vi "GNSS1-SET-5.vi"(4 "DigNum引用句柄 3":refnum<vi>, 6 "Clust引用句柄 2":refnum<vi>, 7 "DigNum引用句柄":refnum<vi>, 9 "DigNum引用句柄 2":refnum<vi>, 10 "Clust引用句柄":refnum<vi>, 11 "Cluster输入":refnum<vi>) -> (3 "添加的数组":u8[](array[numeric]))   [LabVIEW 2012]
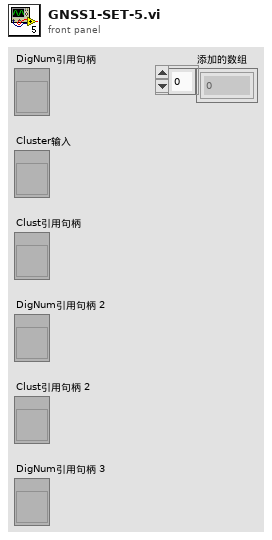
[diagram p1: front panel]
types:
  T1 = cluster{"BD-J2000X轴位置":sgl, "BD-J2000Y轴位置":sgl, "BD-J2000Z轴位置":sgl, "BD-J2000X轴速度":sgl, "BD-J2000Y轴速度":sgl, "BD-J2000Z轴速度":sgl}
  T2 = cluster{"GLOBD-J2000X轴位置":sgl, "GLOBDBD-J2000Y轴位置":sgl, "GLOBD-J2000Z轴位置":sgl, "GLOBD-J2000X轴速度":sgl, "GLOBD-J2000Y轴速度":sgl, "GLOBD-J2000Z轴速度":sgl}
  T3 = cluster{"GPS-J2000X轴位置":sgl, "GPS-J2000Y轴位置":sgl, "GPS-J2000Z轴位置":sgl, "GPS-J2000X轴速度":sgl, "GPS-J2000Y轴速度":sgl, "GPS-J2000Z轴速度":sgl}
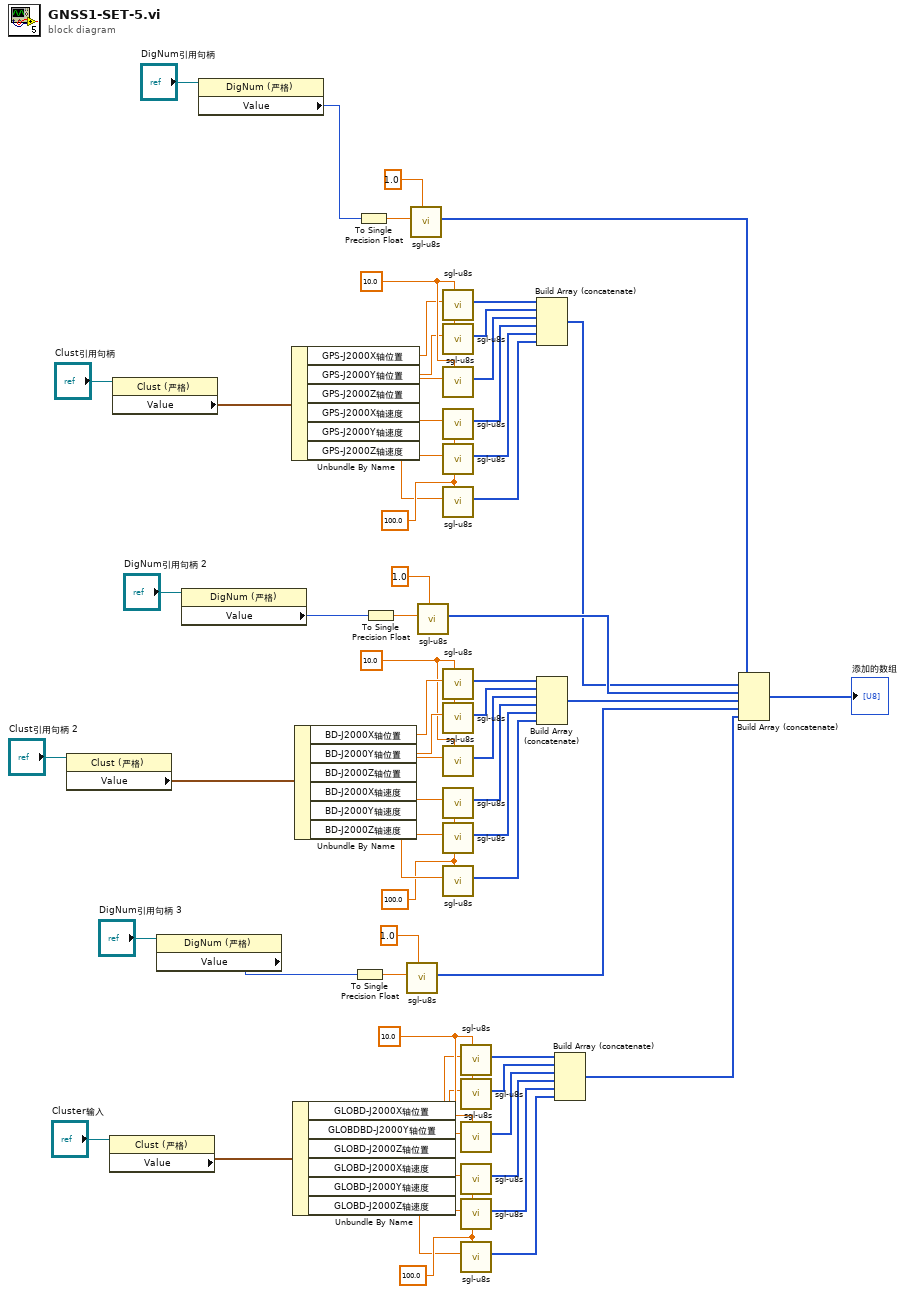
[diagram p0: block diagram]
diagram:
  w58 = sgl 100.0 ("精度")
  w52 = sgl 10.0 ("y")
  w31 = sgl 100.0 ("精度")
  w37 = sgl 10.0 ("y")
  w24 = sgl 100.0 ("精度")
  w18 = sgl 10.0 ("y")
  n1 = property on="属性节点" class="Clust (严格)"(reference="Clust引用句柄 2") -> ("Value"=w59:T1)  [unwired: 1 in, 2 out]
  n2 = property on="属性节点" class="Clust (严格)"(reference="Cluster输入") -> ("Value"=w65:T2)  [unwired: 1 in, 2 out]
  n3 = property on="属性节点" class="Clust (严格)"(reference="Clust引用句柄") -> ("Value"=w25:T3)  [unwired: 1 in, 2 out]
  n4 = property on="属性节点" class="DigNum (严格)"(reference="DigNum引用句柄 3") -> ("Value"=w63:u32)  [unwired: 1 in, 2 out]
  n5 = property on="属性节点" class="DigNum (严格)"(reference="DigNum引用句柄 2") -> ("Value"=w29:u32)  [unwired: 1 in, 2 out]
  n6 = property on="属性节点" class="DigNum (严格)"(reference="DigNum引用句柄") -> ("Value"=w9:u32)  [unwired: 1 in, 2 out]
  n7 = Unbundle By Name(w25) -> ("GPS-J2000X轴位置"=w11:sgl, "GPS-J2000Y轴位置"=w13:sgl, "GPS-J2000Z轴位置"=w14:sgl, "GPS-J2000X轴速度"=w15:sgl, "GPS-J2000Y轴速度"=w16:sgl, "GPS-J2000Z轴速度"=w17:sgl)
  n8 = Unbundle By Name(w65) -> ("GLOBD-J2000X轴位置"=w45:sgl, "GLOBDBD-J2000Y轴位置"=w47:sgl, "GLOBD-J2000Z轴位置"=w48:sgl, "GLOBD-J2000X轴速度"=w49:sgl, "GLOBD-J2000Y轴速度"=w50:sgl, "GLOBD-J2000Z轴速度"=w51:sgl)
  n9 = Unbundle By Name(w59) -> ("BD-J2000X轴位置"=w44:sgl, "BD-J2000Y轴位置"=w42:sgl, "BD-J2000Z轴位置"=w41:sgl, "BD-J2000X轴速度"=w40:sgl, "BD-J2000Y轴速度"=w39:sgl, "BD-J2000Z轴速度"=w38:sgl)
  n10 = To Single Precision Float(number=w63) -> (single precision float=w62:sgl)
  n11 = To Single Precision Float(number=w9) -> (single precision float=w8:sgl)
  n12 = To Single Precision Float(number=w29) -> (single precision float=w27:sgl)
  n13 = call "sgl-u8s.vi"("输入sgl"=w62, "精度"=sgl 1.0) -> ("u8s"=w64:u8[])  [unwired: 8 in]
  n14 = call "sgl-u8s.vi"("输入sgl"=w8, "精度"=sgl 1.0) -> ("u8s"=w10:u8[])  [unwired: 8 in]
  n15 = call "sgl-u8s.vi"("输入sgl"=w27, "精度"=sgl 1.0) -> ("u8s"=w30:u8[])  [unwired: 8 in]
  n16 = call "sgl-u8s.vi"("输入sgl"=w11, "精度"=w18) -> ("u8s"=w12:u8[])  [unwired: 8 in]
  n17 = call "sgl-u8s.vi"("输入sgl"=w13, "精度"=w18) -> ("u8s"=w19:u8[])  [unwired: 8 in]
  n18 = call "sgl-u8s.vi"("输入sgl"=w14, "精度"=w18) -> ("u8s"=w20:u8[])  [unwired: 8 in]
  n19 = call "sgl-u8s.vi"("输入sgl"=w15, "精度"=w24) -> ("u8s"=w21:u8[])  [unwired: 8 in]
  n20 = call "sgl-u8s.vi"("输入sgl"=w16, "精度"=w24) -> ("u8s"=w22:u8[])  [unwired: 8 in]
  n21 = call "sgl-u8s.vi"("输入sgl"=w17, "精度"=w24) -> ("u8s"=w23:u8[])  [unwired: 8 in]
  n22 = call "sgl-u8s.vi"("输入sgl"=w44, "精度"=w37) -> ("u8s"=w43:u8[])  [unwired: 8 in]
  n23 = call "sgl-u8s.vi"("输入sgl"=w42, "精度"=w37) -> ("u8s"=w36:u8[])  [unwired: 8 in]
  n24 = call "sgl-u8s.vi"("输入sgl"=w41, "精度"=w37) -> ("u8s"=w35:u8[])  [unwired: 8 in]
  n25 = call "sgl-u8s.vi"("输入sgl"=w40, "精度"=w31) -> ("u8s"=w34:u8[])  [unwired: 8 in]
  n26 = call "sgl-u8s.vi"("输入sgl"=w39, "精度"=w31) -> ("u8s"=w33:u8[])  [unwired: 8 in]
  n27 = call "sgl-u8s.vi"("输入sgl"=w38, "精度"=w31) -> ("u8s"=w32:u8[])  [unwired: 8 in]
  n28 = call "sgl-u8s.vi"("输入sgl"=w45, "精度"=w52) -> ("u8s"=w46:u8[])  [unwired: 8 in]
  n29 = call "sgl-u8s.vi"("输入sgl"=w47, "精度"=w52) -> ("u8s"=w53:u8[])  [unwired: 8 in]
  n30 = call "sgl-u8s.vi"("输入sgl"=w48, "精度"=w52) -> ("u8s"=w54:u8[])  [unwired: 8 in]
  n31 = call "sgl-u8s.vi"("输入sgl"=w49, "精度"=w58) -> ("u8s"=w55:u8[])  [unwired: 8 in]
  n32 = call "sgl-u8s.vi"("输入sgl"=w50, "精度"=w58) -> ("u8s"=w56:u8[])  [unwired: 8 in]
  n33 = call "sgl-u8s.vi"("输入sgl"=w51, "精度"=w58) -> ("u8s"=w57:u8[])  [unwired: 8 in]
  n34 = Build Array (concatenate)(w12, w19, w20, w21, w22, w23) -> (w26:u8[])
  n35 = Build Array (concatenate)(w43, w36, w35, w34, w33, w32) -> (w60:u8[])
  n36 = Build Array (concatenate)(w46, w53, w54, w55, w56, w57) -> (w66:u8[])
  n37 = Build Array (concatenate)(w10, w26, w30, w60, w64, w66) -> (→"添加的数组":u8[])
